vi "Rotation2d_Div.vi"(9 "Scalar":dbl, 11 "in ROTATION":T1 {"SIN" format="%13.4f"; "COS" format="%13.4f"; "VALUE" format="%13.4f"}) -> (3 "out ROTATION":T1 {"SIN" format="%13.4f"; "COS" format="%13.4f"; "VALUE" format="%13.4f"})   [LabVIEW 2019, in "Trajectory_Library.lvlib"]
doc: "Divides the current rotation (angle) by a scalar.\n\nParameters: \n- IN ROTATION - This ROTATION data structure\n- SCALAR - The value to divide the rotation by.\n\nReturns:\n - OUT ROTATION - THe new ROTATION data structure."
uses:
  Trajectory_Library.lvlib
  TypeDef/ROTATION2D.ctl
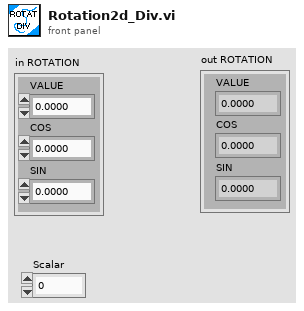
[diagram p1: front panel]
types:
  T1 = typedef "Trajectory_Library.lvlib/ROTATION2D.ctl" = cluster{"VALUE":dbl, "COS":dbl, "SIN":dbl}
  T2 = typedef "WPILib_Math.lvlib/ROTATION2D.ctl" = cluster{"VALUE":dbl, "COS":dbl, "SIN":dbl}
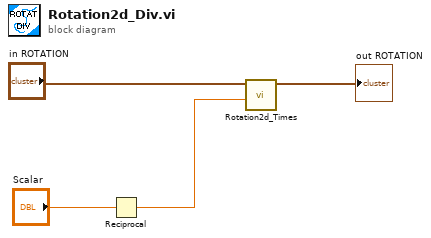
[diagram p0: block diagram]
diagram:
  n1 = Reciprocal(x="Scalar") -> (1/x=w2:dbl)
  n2 = call "Rotation2d_Times.vi"("Scalar"=w2, "in ROTATION"="in ROTATION") -> ("out ROTATION"=→"out ROTATION":T2)  [unwired: 9 in]
